vi "Inline Spawn Root.vi"(4 "UID":string, 6 "Core Actors":refnum<class "Actor.lvclass">[](array[class]), 9 "Mid Actors":refnum<class "Actor.lvclass">[](array[class]), 10 "Edge Actors":refnum<class "Actor.lvclass">[](array[class])) -> (0 "Error out":errorcluster, 5 "Actor out":refnum<class "Actor.lvclass">)   [LabVIEW 2020, in "jettl.lvlib"]
uses:
  jettl.lvlib
  Actor/Actor.lvclass
  Async Elements/Async Elements.lvclass
  Transport/Transport.lvclass
  Attributes/Attributes.lvclass
  Msg/Msg.lvclass
  Base Attributes/Base Attributes/Base Attributes.lvclass
  Base Attributes/Base Attributes.lvlib
  Msgs.ctl
  Attributes.ctl
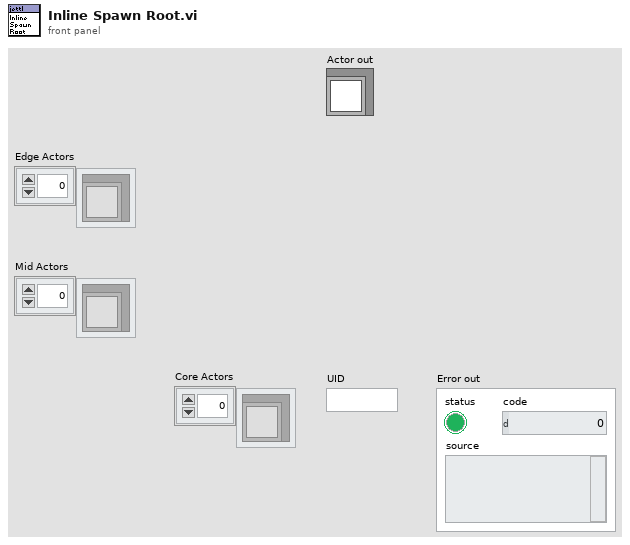
[diagram p1: front panel]
types:
  T1 = typedef "jettl.lvlib/Attributes.ctl" = cluster{"Unified Msgs":T2, "Edge Actors":refnum<class "Actor.lvclass">[], "Core Actors":refnum<class "Actor.lvclass">[], "Parent Attributes":refnum<class "Attributes.lvclass">, "Root":bool, "App Ref":refnum<vi>, "UID":string, "Transport":refnum<class "Transport.lvclass">, "VI Ref":refnum<vi>, "Actors":refnum<class "Actor.lvclass">[]}
  T2 = typedef "jettl.lvlib/Msgs.ctl" = set{refnum<class "Msg.lvclass">}
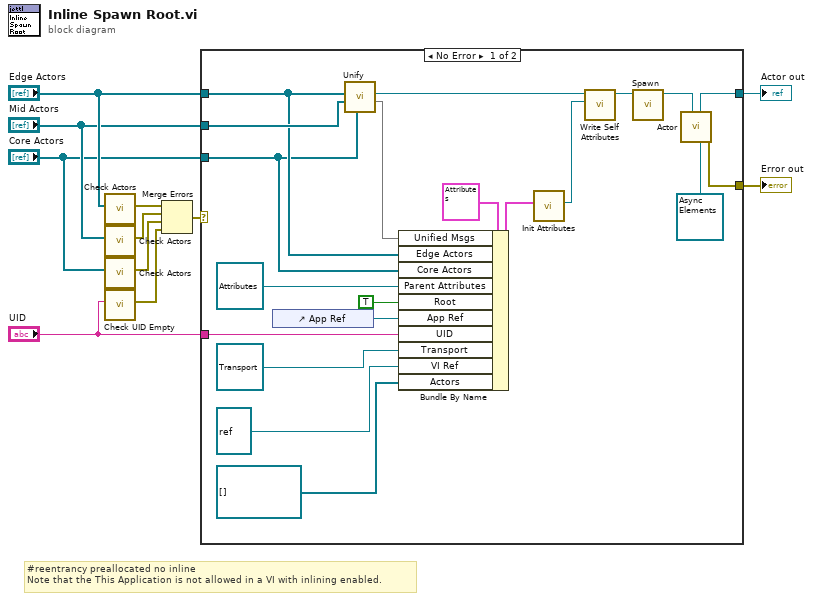
[diagram p0: block diagram]
diagram:
  # "#reentrancy preallocated no inline\nNote that the This Application is not allowed in a VI with inlining enabled."
  n1 = call "Check Actors.vi"("Actors"="Edge Actors") -> ("Error"=w6:errorcluster)  [unwired: 10 in]
  n2 = call "Check Actors.vi"("Actors"="Mid Actors") -> ("Error"=w8:errorcluster)  [unwired: 10 in]
  n3 = call "Check Actors.vi"("Actors"="Core Actors") -> ("Error"=w1:errorcluster)  [unwired: 10 in]
  n4 = call "Check UID Empty.vi"("UID"="UID") -> ("Error"=w7:errorcluster)  [unwired: 10 in]
  n5 = Merge Errors(w6, w8, w1, w7) -> (w9:errorcluster)
  n6 = case shown="No Error" w9 {
    selector: w9 -> [_ w32]
    tunnel: [w18 _] -> w11
    tunnel: [w19 w32] -> w10
    tunnel: "Edge Actors" -> [w15 _]
    tunnel: "UID" -> [w25 _]
    tunnel: "Mid Actors" -> [w16 _]
    tunnel: "Core Actors" -> [w14 _]
    frame No Error {
      n7 = control-ref of="App Ref"() -> (w30:refnum<vi>)
      n8 = call "Unify.vi"("Core Actors"=w14, "Mid Actors"=w16, "Edge Actors"=w15) -> ("Unified Msgs"=w12:T2, "Unified Actor"=w13:refnum<class "Actor.lvclass">)  [unwired: 7 in]
      n9 = Bundle By Name(cluster=T1 {"Unified Msgs"={}, "Edge Actors"=[], "Core Actors"=[], "Parent Attributes"=refnum, "Root"=FALSE, "App Ref"=refnum, "UID"="", "Transport"=refnum, "VI Ref"=refnum, "Actors"=[]} ("Attributes"), "Unified Msgs"=w12, "Edge Actors"=w15, "Core Actors"=w14, "Parent Attributes"=refnum<class "Attributes.lvclass"> refnum, "Root"=TRUE, "App Ref"=w30, "UID"=w25, "Transport"=refnum<class "Transport.lvclass"> refnum, "VI Ref"=refnum<vi> refnum ("Actor Ref"), "Actors"=refnum<class "Actor.lvclass">[] []) -> (w22:T1)
      n10 = call "Init Attributes.vi"("Attributes"=w22) -> ("Attributes"=w31:refnum<class "Attributes.lvclass">)  [unwired: 10 in]
      n11 = call-dynamic "Write Self Attributes.vi"("Self Attributes"=w31, "Actor in"=w13) -> ("Actor out"=w21:refnum<class "Actor.lvclass">)  [unwired: 9 in]
      n12 = call-dynamic "Spawn.vi"("Actor in"=w21) -> ("Actor out"=w17:refnum<class "Actor.lvclass">)  [unwired: 10 in]
      n13 = call "Actor.vi"("Async Elements"=refnum<class "Async Elements.lvclass"> refnum, "Actor in"=w17) -> ("Error out"=w19:errorcluster, "Actor out"=w18:refnum<class "Actor.lvclass">)  [unwired: 8 in]
    }
    frame Error {
    }
  }
  "Error out" <- w10
  "Actor out" <- w11
